vi "LCDSetCursor.vi"(8 "error in (no error)":errorcluster, 9 "Row":u8, 10 "Col":u8, 11 "LCDRef":T1) -> (0 "error out":errorcluster)   [LabVIEW 2013]
uses:
  LCDRef.ctl
  <vilib>/Rock Robotics/WPI/SerialPort/WPI_SerialPortRef.ctl
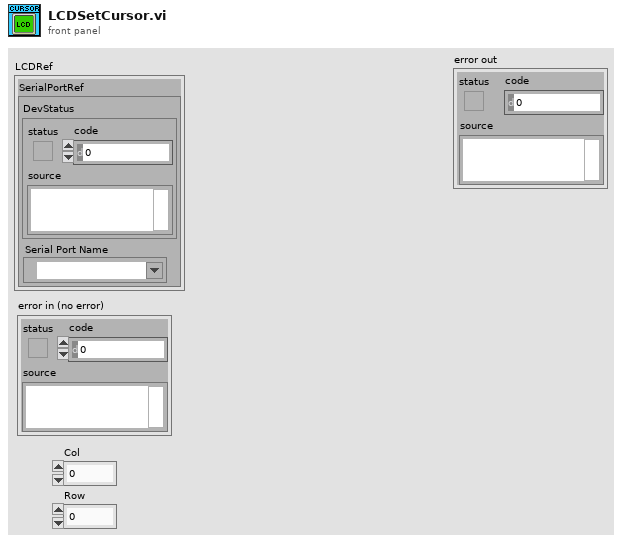
[diagram p1: front panel]
types:
  T1 = typedef "LCDRef.ctl" = cluster{"SerialPortRef":T2}
  T2 = typedef "WPI_SerialPortRef.ctl" = cluster{"DevStatus":errorcluster, "Serial Port Name":refnum<visa-resource-name>}
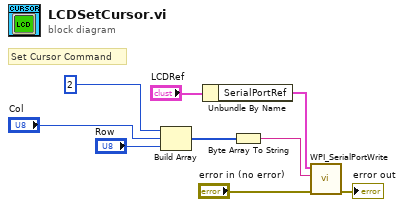
[diagram p0: block diagram]
diagram:
  # "Set Cursor Command"
  n1 = Build Array(u8 2 ("element"), "Col", "Row") -> (w3:u8[])
  n2 = Unbundle By Name("LCDRef") -> ("SerialPortRef"=w1:T2)
  n3 = Byte Array To String(unsigned byte array=w3) -> (string=w4:string)
  n4 = call <vilib>:"WPI_SerialPortWrite.vi"("error in (no error)"="error in (no error)", "Buffer"=w4, "SerialPortRef"=w1) -> ("error out"=→"error out":errorcluster)  [unwired: 6 in, 2 out]
